vi "OPERATEURV2.vi"(8 "errin":errorcluster, 11 "IN":string) -> (0 "error out":errorcluster caption="errout", 3 "Dataout":string)   [LabVIEW 2020]
uses:
  C:/Users/elhajj/OneDrive - FORSEE POWER/Bureau/Support banc de test/Ligne ZENPLUS/Code LabVIEW/CODE/02 SLIM ZEN WS 500/SubVi/FGV.ctl
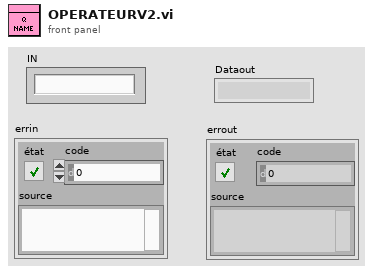
[diagram p1: front panel]
types:
  T1 = typedef "FGV.ctl" = enum16{"GET", "SET", "RAZ"}
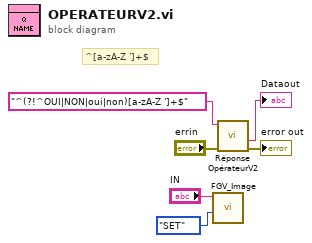
[diagram p0: block diagram]
diagram:
  # "^[a-zA-Z ']+$"
  n1 = call "FGV_Image.vi"("Énum"=FGV."SET", "IN"="IN") -> ()  [unwired: 9 in, 1 out]
  n2 = call "Réponse OpérateurV2.vi"("errin"="errin", "expression régulière"="^(?!^OUI|NON|oui|non)[a-zA-Z ']+$") -> ("errout"=→"error out":errorcluster, "toute l'expression"=→"Dataout":string)  [unwired: 7 in, 1 out]
